vi "Pointcloud Update Meshes.vi"(8 "error in (no error)":errorcluster, 10 "2D Map":dbl[][](array[numeric]), 11 "Pointcloud in":refnum<class "Pointcloud.lvclass">) -> (0 "error out":errorcluster, 3 "Pointcloud out":refnum<class "Pointcloud.lvclass">)   [LabVIEW 2018, in "Pointcloud.lvclass"]
uses:
  Pointcloud.lvclass
  Pointcloud.lvclass/Pointcloud.ctl
  <vilib>/Utility/miscctls.llb/LVRGBAColorTypeDef.ctl
  <vilib>/picture/3D Picture Control/NI_3D Picture Control.lvlib
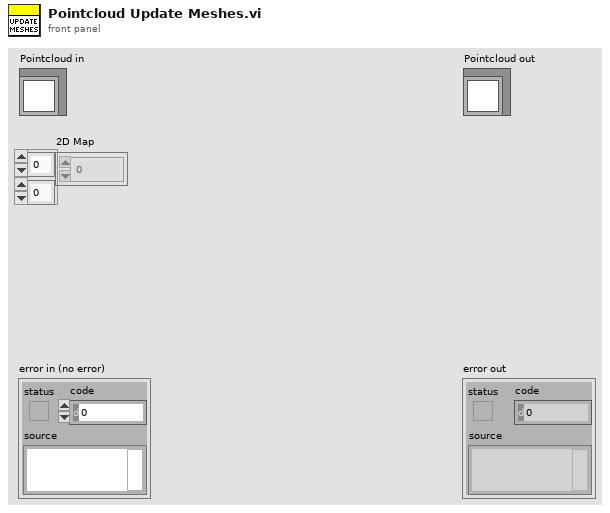
[diagram p1: front panel]
types:
  T1 = typedef "LVRGBAColorTypeDef.ctl" = cluster{"Red":sgl, "Green":sgl, "Blue":sgl, "Alpha":sgl}
  T2 = enum16{"Overall", "Per Primitive", "Per Vertex", "Binding Off"}
  T3 = enum16{"Points", "Lines", "Line Strip", "Line Loop", "Triangles", "Triangle Strip", "Triangle Fan", "Quads", "Quad Strip", "Polygon"}
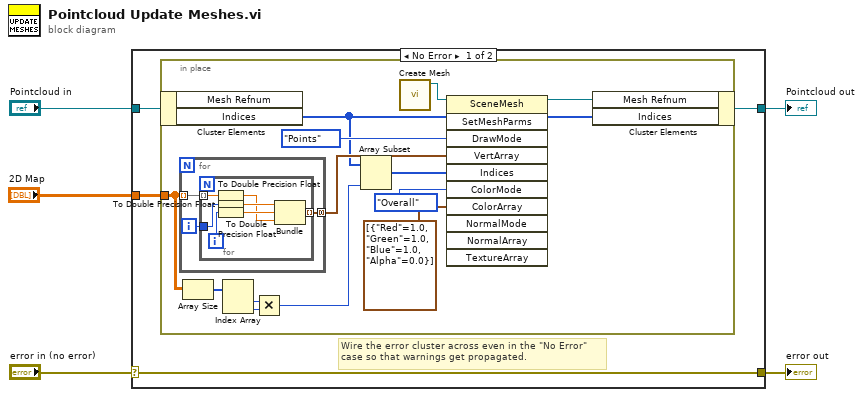
[diagram p0: block diagram]
diagram:
  n1 = case shown="No Error" "error in (no error)" {
    selector: "error in (no error)" -> [w9 w34]
    tunnel: [w9 w34] -> w4
    tunnel: [w7 w33] -> w2
    tunnel: "Pointcloud in" -> [w8 w33]
    tunnel: "2D Map" -> [w6 _]
    frame No Error {
      # "Wire the error cluster across even in the \"No Error\"\ncase so that warnings get propagated."
      n2 = in-place {
        in-place-border: w6 -> [w15]
        n3 = in-place-cluster #1(w8) -> ("Indices"=w19:i32[])  [unwired: 1 out]
        n4 = for {
          tunnel: w15 -> [w25] mode=indexing
          tunnel: [w23] -> w20 mode=concatenating
          i -> [w24]
          n5 = for {
            tunnel: w25 -> [w32] mode=indexing
            tunnel: w24 -> [w26]
            tunnel: [w28] -> w23 mode=indexing
            i -> [w27]
            n6 = To Double Precision Float(number=w32) -> (double precision float=w29:dbl)
            n7 = To Double Precision Float(number=w26) -> (double precision float=w31:dbl)
            n8 = To Double Precision Float(number=w27) -> (double precision float=w30:dbl)
            n9 = Bundle(w31, w30, w29) -> (w28:cluster{dbl, dbl, dbl})  [unwired: 1 in]
          }
        }
        n10 = Array Size(array=w15) -> (size(s)=w14:i32[])
        n11 = Index Array(array=w14) -> (element #1=w12:i32, element #2=w13:i32)  [unwired: 2 in]
        n12 = Multiply(x=w12, y=w13) -> (x*y=w11:i32)
        n13 = Array Subset(array=w19, length=w11) -> (w18:i32[])  [unwired: 1 in]
        n14 = call <vilib>:"Create Mesh.vi"() -> ("New Mesh Refnum"=w10:refnum<vi>)  [unwired: 10 in, 1 out]
        n15 = invoke class="SceneMesh" method="SetMeshParms"(reference=w10, "DrawMode"=T3."Points" ("Draw Mode"), "VertArray"=w20, "Indices"=w18, "ColorMode"=T2."Overall" ("Color Binding Mode"), "ColorArray"=T1[] [{"Red"=1.0, "Green"=1.0, "Blue"=1.0, "Alpha"=0.0}] ("Color Array")) -> (reference out=w22:refnum<vi>)  [unwired: 5 in, 10 out]
        n16 = in-place-cluster #1("Mesh Refnum"=w22, "Indices"=w19) -> (w7:refnum<class "Pointcloud.lvclass">)
      }
    }
    frame Error {
    }
  }
  "error out" <- w4
  "Pointcloud out" <- w2
